vi "Contour Line_Search Near Connected Contour Points.vi"(7 "Stack In":bool[](array[boolean]), 10 "search edge":T1, 11 "Intersected Edges":T2(array[cluster])) -> (2 "connected index":i32, 3 "find?":bool, 5 "Stack Out":bool[](array[boolean]))   [LabVIEW 2020, in "NI_AAL_Geometry.lvlib"]
uses:
  <vilib>/Analysis/NI_AAL_Geometry.lvlib
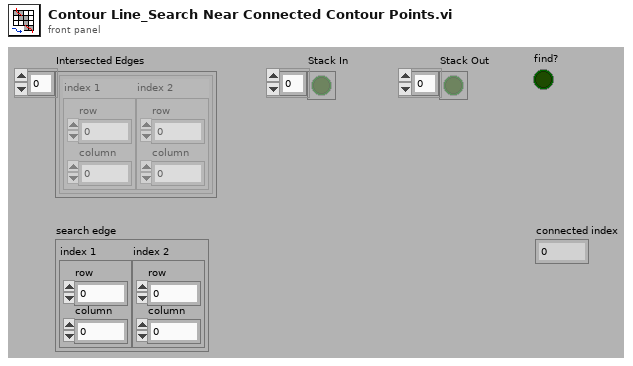
[diagram p1: front panel]
types:
  T1 = cluster{"index 1":cluster{"row":i32, "column":i32}, "index 2":cluster{"row":i32, "column":i32}}
  T2 = cluster{"index 1":cluster{"row":i32, "column":i32}, "index 2":cluster{"row":i32, "column":i32}}[]
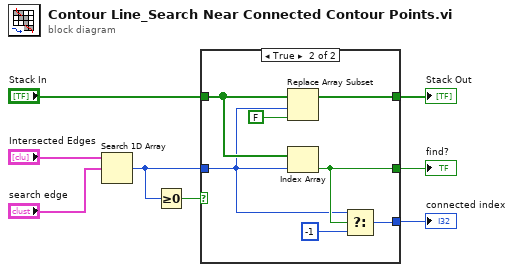
[diagram p0: block diagram]
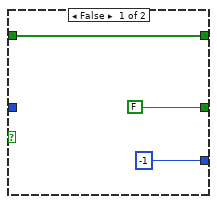
[diagram p2: hidden frame]
diagram:
  n1 = Search 1D Array(1D array="Intersected Edges", element="search edge") -> (index of element=w5:i32)  [unwired: 1 out]
  n2 = Greater Or Equal To 0?(x=w5) -> (x >= 0?=w6:bool)
  n3 = case shown="True" w6 {
    tunnel: w5 -> [_ w13]
    tunnel: "Stack In" -> [w10 w18]
    tunnel: [FALSE ("Boolean") w16] -> w3
    tunnel: [w10 w17] -> w2
    tunnel: [-1 ("f") w14] -> w1
    frame False {
    }
    frame True {
      n4 = Replace Array Subset(array=w18, new element=FALSE ("new element/subarray"), index=w13) -> (w17:bool[])
      n5 = Index Array(array=w18, index=w13) -> (element=w16:bool)
      n6 = Select(t=w13, s=w16, f=-1) -> (s? t:f=w14:i32)
    }
  }
  "Stack Out" <- w2
  "connected index" <- w1
  "find?" <- w3
